vi "Lock-in detector.vi"(4 "Clip units of Ts off":dbl, 5 "Filter type":enum16{"None", "IIR", "FIR"}(ring), 6 "Time constant":dbl=0.0001 format="%#_6p", 7 "Fix time delay":bool=TRUE, 8 "Error In":errorcluster, 9 "Phase":dbl, 10 "Frequency":dbl format="%_19p", 11 "Data in":waveform(dbl)) -> (0 "Error Out":errorcluster, 3 "Data out":waveform(dbl)[](array[waveform]))   [LabVIEW 2015]
uses:
  <vilib>/Waveform/WDTOps.llb/WDT Number of Waveform Samples DBL.vi
  <vilib>/measure/NI_MABase.lvlib
panel:
  out "Waveform Graph":waveform(dbl)[](graph)
  in  "offset":dbl format="%0.2p"
  in  "amplitude":dbl=1.0 format="%0.2p"
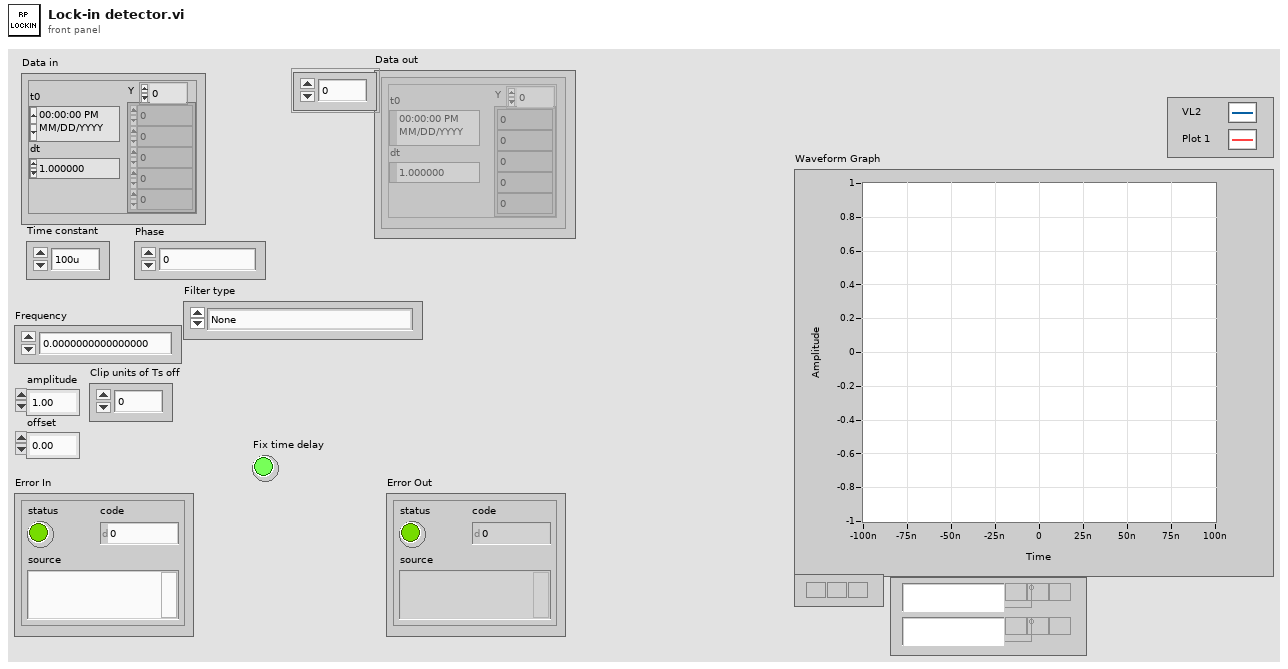
[diagram p1: front panel]
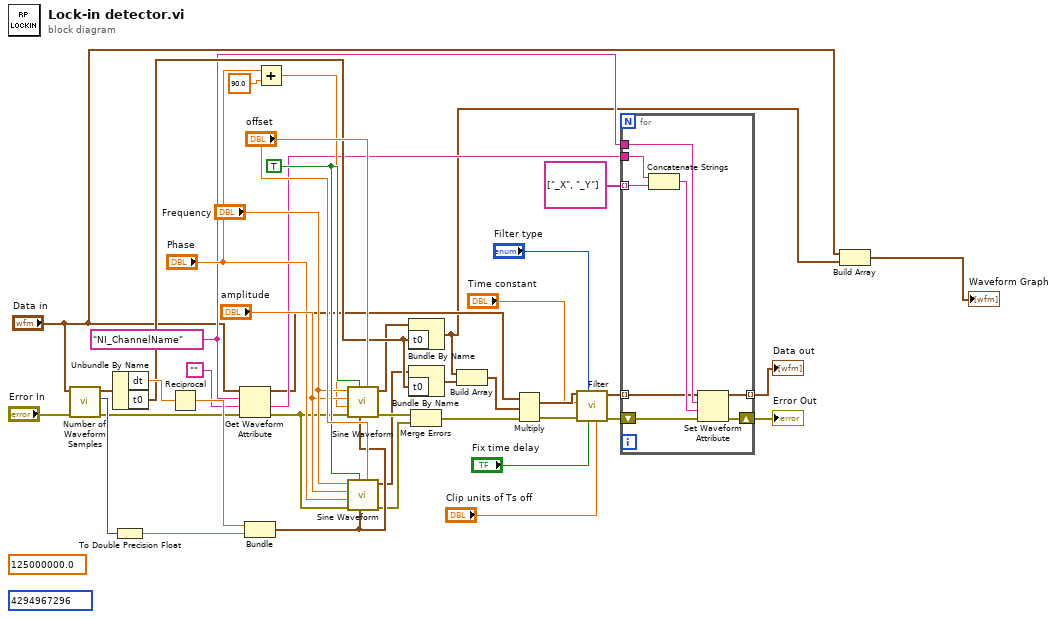
[diagram p0: block diagram]
diagram:
  w15 = "NI_ChannelName" ("name")
  w35 = TRUE ("reset signal")
  (unwired) u64 4294967296
  (unwired) 125000000.0
  n1 = call-poly <vilib>:"Number of Waveform Samples.vi"("error in (no error)"="Error In", "waveform in"="Data in") -> ("error out"=w27:errorcluster, "number of samples"=w41:i32, "waveform out"=w42:waveform(dbl))  [unwired: 7 in]
  n2 = Unbundle By Name(w42) -> ("dt"=w38:dbl, "t0"=w28:timestamp)
  n3 = To Double Precision Float(number=w41) -> (double precision float=w39:dbl)
  n4 = Reciprocal(x=w38) -> (1/x=w40:dbl)
  n5 = Get Waveform Attribute(4:w27, 5:"", 6:w15, 7:"Data in") -> (0:w26:errorcluster, 1:w16:string, 3:w5:waveform(dbl))  [unwired: 1 out]
  n6 = Bundle(w40, w39) -> (w29:cluster{dbl, dbl})  [unwired: 1 in]
  n7 = Add(x="Phase", y=90.0) -> (x+y=w31:dbl)
  n8 = call <vilib>:"Sine Waveform.vi"("offset"="offset", "sampling info"=w29, "reset signal"=w35, "error in (no error)"=w26, "phase"=w31, "amplitude"="amplitude", "frequency"="Frequency") -> ("error out"=w10:errorcluster, "signal out"=w3:waveform(dbl))  [unwired: 3 in]
  n9 = call <vilib>:"Sine Waveform.vi"("offset"="offset", "sampling info"=w29, "reset signal"=w35, "error in (no error)"=w26, "phase"="Phase", "amplitude"="amplitude", "frequency"="Frequency") -> ("error out"=w9:errorcluster, "signal out"=w7:waveform(dbl))  [unwired: 3 in]
  n10 = Bundle By Name(cluster=w3, "t0"=w28) -> (w1:waveform(dbl))
  n11 = Bundle By Name(cluster=w7, "t0"=w28) -> (w6:waveform(dbl))
  n12 = Merge Errors(w10, w9) -> (w8:errorcluster)
  n13 = Build Array(w1, w6) -> (w24:waveform(dbl)[])
  n14 = Multiply(1:w24, 2:w5, 4:w8) -> (0:w23:waveform(dbl)[], 3:w22:errorcluster)
  n15 = call "Filter.vi"("Clip units of Ts off"="Clip units of Ts off", "Fix time delay"="Fix time delay", "Filter type"="Filter type", "Error In"=w22, "Time constant"="Time constant", "Data"=w23) -> ("Error Out"=w13:errorcluster, "Data out"=w14:waveform(dbl)[])  [unwired: 3 in, 1 out]
  n16 = for {
    tunnel: string[] ["_X", "_Y"] -> [w50] mode=indexing
    tunnel: w16 -> [w49]
    tunnel: w15 -> [w47]
    tunnel: w14 -> [w46] mode=indexing
    tunnel: [w45] -> w12 mode=indexing
    shift-right: [w44] -> w11
    shift-left: w13 -> [w43]
    n17 = Concatenate Strings(w49, w50) -> (w48:string)
    n18 = Set Waveform Attribute(4:w43, 5:w48, 6:w47, 7:w46) -> (0:w44:errorcluster, 3:w45:waveform(dbl))  [unwired: 1 out]
  }
  "Error Out" <- w11
  "Data out" <- w12
  n19 = Build Array("Data in", w1) -> (→"Waveform Graph":waveform(dbl)[])
